vi "BuildPresentWorld.vi"() -> (2 "Valid slides?":bool, 3 "SlideInfo":T1[](array[typedef]), 4 "Scene.Object Out":refnum<vi>)   [LabVIEW 2010]
uses:
  SlideTypeDef.ctl
  <vilib>/Utility/file.llb/Read From Spreadsheet File (string).vi
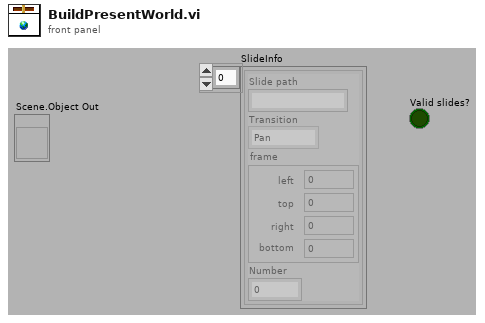
[diagram p1: front panel]
types:
  T1 = typedef "SlideTypeDef.ctl" = cluster{"Slide path":string, "Transition":enum16{"Pan", "Zoom-pan-zoom", "Zoom-wait-Zoom"}, "frame":cluster{"left":i16, "top":i16, "right":i16, "bottom":i16}, "Number":i32}
  T2 = typedef "ParamterCluster.ctl" = cluster{"bounce?":bool, "black?":bool, "slide number":i32, "hide?":bool, "selection":bool}
  T3 = cluster{string, "Transition":enum16{"Pan", "Zoom-pan-zoom"}, cluster{sgl, sgl, "y":dbl, "y":dbl}, "slide number":i32}
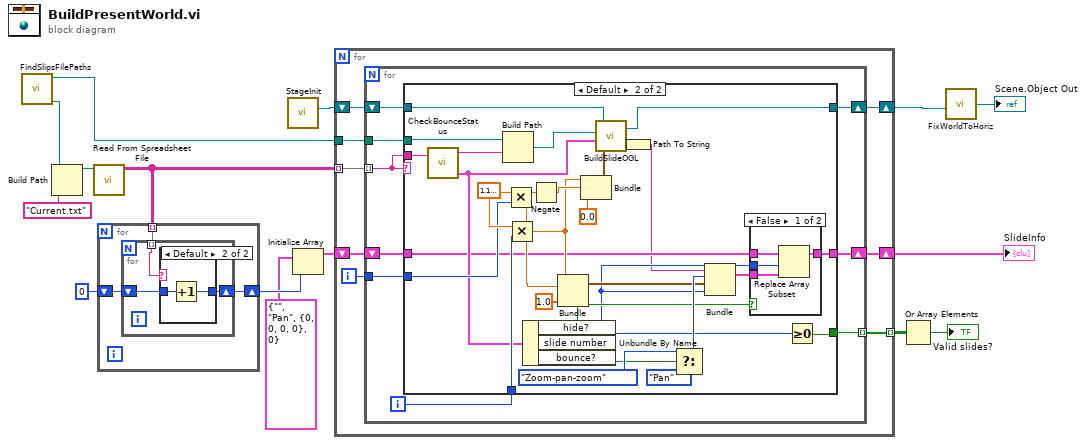
[diagram p0: block diagram]
diagram:
  n1 = call "FindSlipsFilePaths.vi"() -> ("Playlists"=w2:path, "Slides"=w1:path)  [unwired: 2 in, 3 out]
  n2 = Build Path(base path=w2, name or relative path="Current.txt") -> (appended path=w10:path)
  n3 = call-poly <vilib>:"Read From Spreadsheet File.vi"("file path (dialog if empty)"=w10) -> ("all rows"=w9:string[][])  [unwired: 6 in, 4 out]
  n4 = for {
    tunnel: w9 -> [w18] mode=indexing
    shift-right: [w17] -> w7
    shift-left: 0 -> [w16]
    n5 = for {
      tunnel: w18 -> [w21] mode=indexing
      shift-right: [w20] -> w17
      shift-left: w16 -> [w19]
      n6 = case shown="Default" w21 {
        tunnel: [w22 w24] -> w20
        tunnel: w19 -> [w22 w23]
        frame "" {
        }
        frame Default {
          n7 = Increment(x=w23) -> (x+1=w24:i32)
        }
      }
    }
  }
  n8 = call <userlib>:"StageInit.vi"() -> ("Stage out"=w13:refnum<vi>)  [unwired: 4 in, 1 out]
  n9 = Initialize Array(T1 {"Slide path"="", "Transition"=enum."Pan", "frame"={"left"=0, "top"=0, "right"=0, "bottom"=0}, "Number"=0}, w7) -> (w6:T1[])
  n10 = for {
    shift-right: [w31] -> w14
    shift-left: w13 -> [w32]
    tunnel: w9 -> [w30] mode=indexing
    tunnel: w1 -> [w29]
    shift-right: [w27] -> w12
    shift-left: w6 -> [w26]
    tunnel: [w25] -> w4 mode=indexing
    i -> [w28]
    n11 = for {
      shift-right: [w40] -> w31
      shift-left: w32 -> [w41]
      tunnel: w29 -> [w39]
      tunnel: w30 -> [w36] mode=indexing
      tunnel: w28 -> [w38]
      shift-right: [w35] -> w27
      shift-left: w26 -> [w34]
      tunnel: [w33] -> w25 mode=indexing
      i -> [w37]
      n12 = case shown="Default" w36 {
        tunnel: w41 -> [w43 w72]
        tunnel: [w43 w71] -> w40
        tunnel: w39 -> [_ w69]
        tunnel: w36 -> [_ w55]
        tunnel: w38 -> [_ w57]
        tunnel: w37 -> [_ w56]
        tunnel: [w42 w50] -> w35
        tunnel: w34 -> [w42 w51]
        tunnel: [_ w46] -> w33
        frame "" {
        }
        frame Default {
          w44 = 1.0 ("y")
          w67 = sgl 1.1 ("Final Position")
          n13 = call "CheckBounceStatus.vi"("File Name"=w55) -> ("Parameters"=w53:T2, "file name"=w54:string)  [unwired: 1 in, 1 out]
          n14 = Build Path(base path=w69, name or relative path=w54) -> (appended path=w68:path)
          n15 = Multiply(x=w67, y=w57) -> (x*y=w60:sgl)
          n16 = Multiply(x=w67, y=w56) -> (x*y=w61:sgl)
          n17 = Unbundle By Name(w53) -> ("hide?"=w48:bool, "slide number"=w47:i32, "bounce?"=w52:bool)
          n18 = Negate(x=w60) -> (-x=w65:sgl)
          n19 = Bundle(w61, w60, "y"=w44, "y"=w44) -> (w58:cluster{sgl, sgl, "y":dbl, "y":dbl})  [unwired: 1 in]
          n20 = Bundle(w61, w65, "y"=0.0) -> (w70:cluster{sgl, sgl, "y":dbl})  [unwired: 1 in]
          n21 = call "BuildSlideOGL.vi"("Translation"=w70, "Parameters"=w53, "slide"=w68, "Stage In"=w72) -> ("Slide path"=w64:path, "Stage out"=w71:refnum<vi>)
          n22 = Path To String(path=w64) -> (string=w45:string)
          n23 = Select(t=enum16{"Pan", "Zoom-pan-zoom"}."Zoom-pan-zoom" ("Transition"), s=w52, f=enum16{"Pan", "Zoom-pan-zoom"}."Pan" ("Transition")) -> (s? t:f=w59:enum16{"Pan", "Zoom-pan-zoom"})
          n24 = Bundle(w45, "Transition"=w59, w58, "slide number"=w47) -> (w49:T3)  [unwired: 1 in]
          n25 = case shown="False" w48 {
            tunnel: w51 -> [w76 w77]
            tunnel: [w75 w77] -> w50
            tunnel: w49 -> [w73 _]
            tunnel: w47 -> [w74 _]
            frame False {
              n26 = Replace Array Subset(array=w76, new element=w73, index=w74) -> (w75:T1[])
            }
            frame True {
            }
          }
          n27 = Greater Or Equal To 0?(x=w47) -> (x >= 0?=w46:bool)
        }
      }
    }
  }
  "SlideInfo" <- w12
  n28 = Or Array Elements(Boolean array=w4) -> (logical OR=→"Valid slides?":bool)
  n29 = call "FixWorldToHoriz.vi"("Stage In"=w14) -> ("Scene.Object Out"=→"Scene.Object Out":refnum<vi>)
